vi "Rename Frame.vi"(8 "error in (no error)":errorcluster, 9 "New Frame Name (with quotes)":string, 10 "Old Frame Name (with quotes)":string, 11 "JKI SM in":refnum<class "JKI SM.lvclass">) -> (0 "error out":errorcluster, 3 "JKI SM out":refnum<class "JKI SM.lvclass">)   [LabVIEW 2020, in "JKI State Machine API.lvlib" / "JKI SM.lvclass"]
uses:
  JKI SM.lvclass
  JKI SM.lvclass/JKI SM.ctl
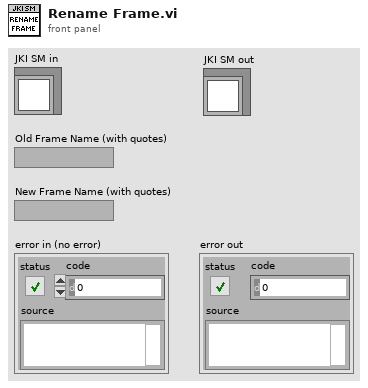
[diagram p1: front panel]
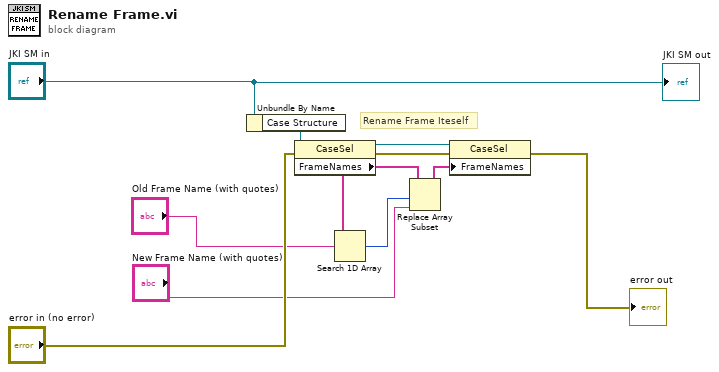
[diagram p0: block diagram]
diagram:
  # "Rename Frame Iteself"
  n1 = Unbundle By Name("JKI SM in") -> ("Case Structure"=w2:refnum<vi>)
  n2 = property class="CaseSel"(reference=w2, error in="error in (no error)") -> (reference out=w3:refnum<vi>, error out=w4:errorcluster, "FrameNames"=w7:string[])
  n3 = Search 1D Array(1D array=w7, element="Old Frame Name (with quotes)") -> (index of element=w10:i32)  [unwired: 1 in]
  n4 = Replace Array Subset(array=w7, new element="New Frame Name (with quotes)", index=w10) -> (w5:string[])
  n5 = property class="CaseSel"(reference=w3, error in=w4, "FrameNames"=w5) -> (error out=→"error out":errorcluster)  [unwired: 1 out]
  "JKI SM out" <- "JKI SM in"
